vi "HW_GEN - DAQ Queue Names Management.vi"(7 "Oper.":T1=enum."ReadName", 9 "error in":errorcluster caption="错误输入", 10 "Qname in":string) -> (1 "error out":errorcluster caption="错误输出", 2 "DAQ Q Names[]":string[](array[string]))   [LabVIEW 2016]
uses:
  Ctrls/HardWare Gen _ DAQ Queue Names FGV Operations.ctl
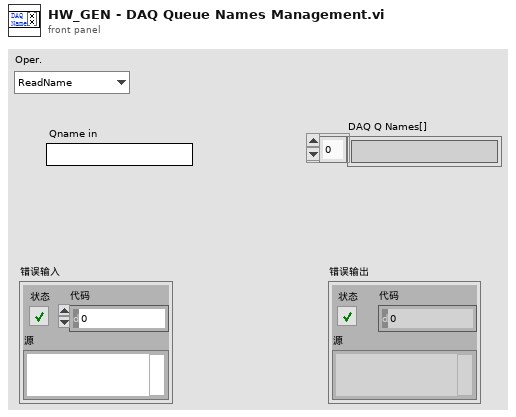
[diagram p1: front panel]
types:
  T1 = typedef "HardWare Gen _ DAQ Queue Names FGV Operations.ctl" = enum16{"Initialize", "AddName", "ReadName"}
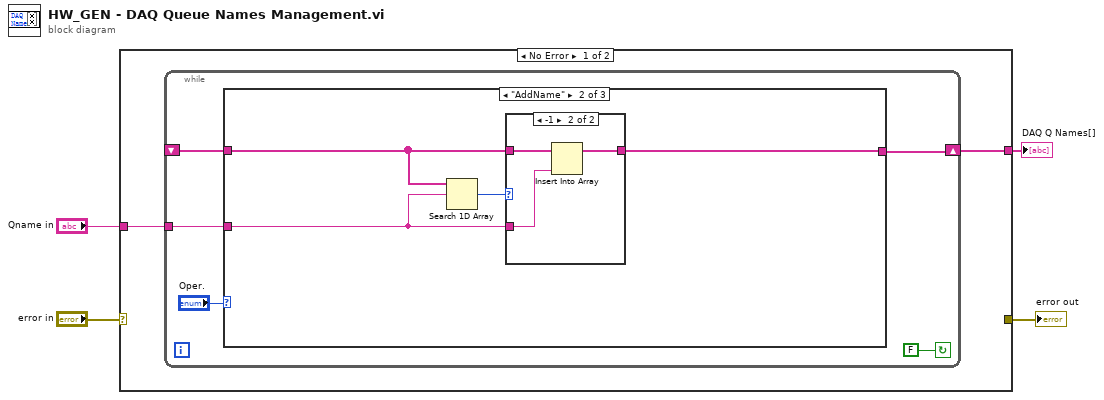
[diagram p0: block diagram]
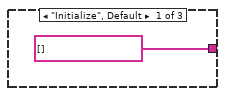
[diagram p2: hidden frame]
diagram:
  n1 = case shown="No Error" "error in" {
    selector: "error in" -> [_ w22]
    tunnel: [_ w22] -> w3
    tunnel: [w6 _] -> w2
    tunnel: "Qname in" -> [w5 _]
    frame No Error {
      n2 = while {
        tunnel: w5 -> [w8]
        shift-right: [w9] -> w6
        shift-left: _ -> [w7]
        stop <- FALSE continue-if-true
        n3 = case shown="\"AddName\"" "Oper." {
          tunnel: [string[] [] w14 w21] -> w9
          tunnel: w8 -> [_ w16 _]
          tunnel: w7 -> [_ w15 w21]
          frame "Initialize", Default {
          }
          frame "AddName" {
            n4 = Search 1D Array(1D array=w15, element=w16) -> (index of element=w13:i32)  [unwired: 1 in]
            n5 = case shown="-1" w13 {
              tunnel: w15 -> [w17 w20]
              tunnel: [w17 w19] -> w14
              tunnel: w16 -> [_ w18]
              frame 0, Default {
              }
              frame -1 {
                n6 = Insert Into Array(array=w20, new element=w18) -> (w19:string[])  [unwired: 1 in]
              }
            }
          }
          frame "ReadName" {
          }
        }
      }
    }
    frame Error {
    }
  }
  "error out" <- w3
  "DAQ Q Names[]" <- w2
